vi "Launch Animation Actor.vi"(8 "error in (no error)":errorcluster, 11 "Controller in":refnum<class "Controller.lvclass">) -> (0 "error out":errorcluster, 3 "Controller out":refnum<class "Controller.lvclass">)   [LabVIEW 2024, in "Controller.lvlib" / "Controller.lvclass"]
uses:
  Controller.lvclass
  C:/Program Files/National Instruments/LabVIEW 2024/vi.lib/ActorFramework/Actor/Actor.lvclass
  Grid Animation/Grid Animation/Grid Animation.lvclass
  Controller.lvclass/Controller.ctl
  Grid Animation/Grid Animation/Grid Animation.lvclass/Grid Animation.ctl
  <vilib>/ActorFramework/Message Enqueuer/Message Enqueuer.lvclass/Message Enqueuer.ctl
  Grid Animation/Grid Animation/Write Grid Actor's Enquerer.vi
  Grid Animation/Grid Animation/Write MC's Grid.vi
  <vilib>/ActorFramework/Message Enqueuer/Enqueue.vi
  <vilib>/ActorFramework/Stop Msg/Stop Msg.lvclass
  C:/Program Files/National Instruments/LabVIEW 2024/vi.lib/ActorFramework/Message/Message.lvclass
  <vilib>/ActorFramework/Message Priority Queue/Priority Enqueue.vi
  <vilib>/ActorFramework/Actor/Actor.lvclass
  C:/Users/ekerry/challenge-of-champions/Grid Animation/Grid Animation/Grid Animation.lvclass
  C:/Users/ekerry/challenge-of-champions/Controller/Controller/Controller.lvclass
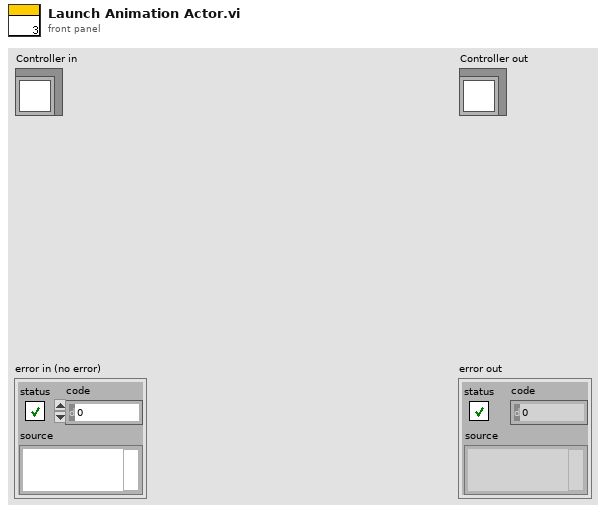
[diagram p1: front panel]
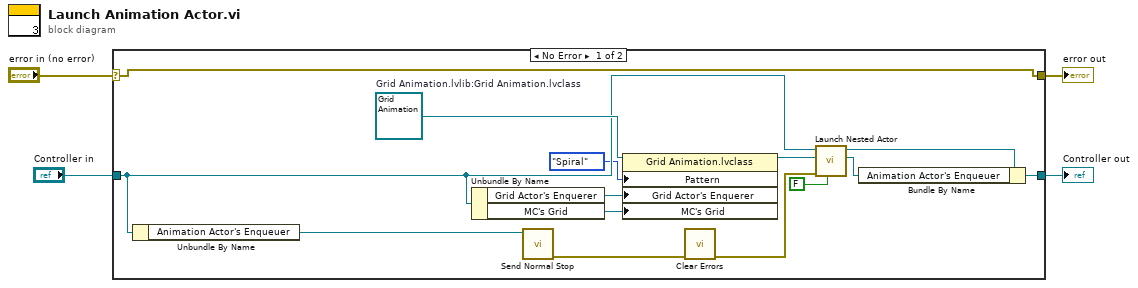
[diagram p0: block diagram]
diagram:
  n1 = case shown="No Error" "error in (no error)" {
    selector: "error in (no error)" -> [w18 w20]
    tunnel: [w18 w20] -> w3
    tunnel: [w10 w19] -> w1
    tunnel: "Controller in" -> [w9 w19]
    frame No Error {
      w17 = refnum<class "Grid Animation.lvclass"> refnum  # Grid Animation.lvlib:Grid Animation.lvclass
      n2 = Unbundle By Name(w9) -> ("Animation Actor's Enqueuer"=w8:refnum<class "Message Enqueuer.lvclass">)
      n3 = Unbundle By Name(w9) -> ("Grid Actor's Enquerer"=w15:refnum<class "Message Enqueuer.lvclass">, "MC's Grid"=w14:refnum<class "Message Enqueuer.lvclass">)
      n4 = call <vilib>:"Send Normal Stop.vi"("Message Enqueuer"=w8) -> ("error out"=w7:errorcluster)  [unwired: 10 in]
      n5 = property class="Grid Animation.lvclass"(reference=w17, "Pattern"=enum16{"Rows", "Spiral"}."Spiral", "Grid Actor's Enquerer"=w15, "MC's Grid"=w14) -> (reference out=w16:refnum<class "Grid Animation.lvclass">)  [unwired: 1 in, 1 out]
      n6 = call <vilib>:"Clear Errors.vi"("error in (no error)"=w7) -> ("error out"=w6:errorcluster)  [unwired: 5 in, 1 out]
      n7 = call <vilib>:"Launch Nested Actor.vi"("Open Actor Core front panel? (F)"=FALSE, "error in (no error)"=w6, "Nested Actor"=w16, "Caller Actor in"=w9) -> ("Nested Actor's Enqueuer"=w11:refnum<class "Message Enqueuer.lvclass">, "Caller Actor out"=w12:refnum<class "Controller.lvclass">)  [unwired: 5 in, 1 out]
      n8 = Bundle By Name(cluster=w12, "Animation Actor's Enqueuer"=w11) -> (w10:refnum<class "Controller.lvclass">)
    }
    frame Error {
    }
  }
  "error out" <- w3
  "Controller out" <- w1
